vi "Set FFT Config.vi"(8 "error in (no error)":errorcluster, 9 "Batch Size":u64=100 format="%.0p FFT", 10 "FFT Size":u64=2000000 format="%.0p Samples", 11 "GPU FFT Calculator in":refnum<class "GPU FFT Calculator.lvclass">) -> (0 "error out":errorcluster, 3 "GPU FFT Calculator out":refnum<class "GPU FFT Calculator.lvclass">)   [LabVIEW 2020, in "GPU FFT Calculator.lvlib" / "GPU FFT Calculator.lvclass"]
uses:
  GPU FFT Calculator.lvclass
  GPU FFT Calculator.lvclass/GPU FFT Calculator.ctl
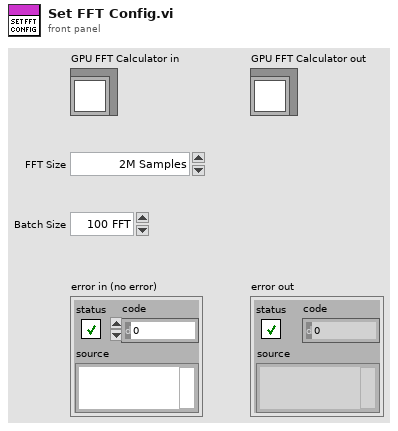
[diagram p1: front panel]
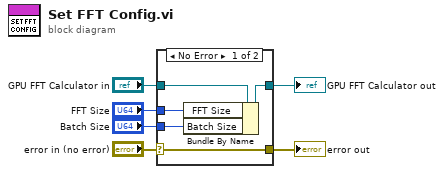
[diagram p0: block diagram]
diagram:
  n1 = case shown="No Error" "error in (no error)" {
    selector: "error in (no error)" -> [w10 w13]
    tunnel: [w10 w13] -> w5
    tunnel: [w9 w12] -> w3
    tunnel: "GPU FFT Calculator in" -> [w11 w12]
    tunnel: "FFT Size" -> [w8 _]
    tunnel: "Batch Size" -> [w7 _]
    frame No Error {
      n2 = Bundle By Name(cluster=w11, "FFT Size"=w8, "Batch Size"=w7) -> (w9:refnum<class "GPU FFT Calculator.lvclass">)
    }
    frame Error {
    }
  }
  "error out" <- w5
  "GPU FFT Calculator out" <- w3
